vi "thcd_visa_init.vi"(2 "err_in":errorcluster, 3 "Serial Settings:Baud Rate":u32(ring)=19200 items=["9.6KHz"=9600, "19.2KHz"=19200], 4 "thcd_visa":refnum<visa-resource-name>) -> (0 "err_out":errorcluster, 1 "thcd_visa":refnum<visa-resource-name>)   [LabVIEW 2018, in "1039_mod.lvlib"]
uses:
  <vilib>/Instr/_visa.llb/VISA Flush IO Buffer Mask.ctl
  1039_mod/1039_mod.lvlib
panel:
  in  "Mask":T1=64 items=["Flush Receive Buffer"=16, "Write Transmit Buffer to Device"=32, "Flush Receive Buffer (No I/O)"=64, "Flush Transmit Buffer"=128]
  in  "Message Based Settings:Suppress End Enable":bool
  in  "Message Based Settings:Send End Enable":bool=TRUE
  in  "Message Based Settings:Termination Character Enable":bool=TRUE
  in  "Serial Settings:End Mode for Writes":u16(ring)=2 items=["None", "Last Bit", "TermChar", "Break"]
  in  "Serial Settings:End Mode for Reads":u16(ring)=2 items=["None", "Last Bit", "TermChar"]
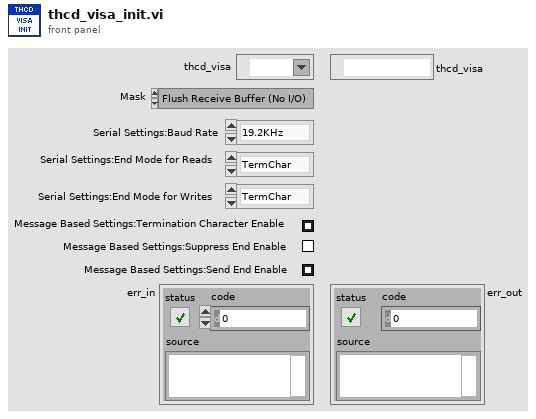
[diagram p1: front panel]
types:
  T1 = typedef "VISA Flush IO Buffer Mask.ctl" = u16
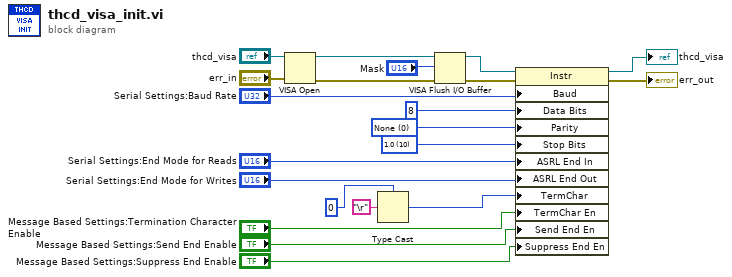
[diagram p0: block diagram]
diagram:
  w18 = u16 10 items=["1.0"=10, "1.5"=15, "2.0"=20] ("Serial Settings:Stop Bits")
  w19 = u16 0 items=["None", "Odd", "Even", "Mark", "Space"] ("Serial Settings:Parity")
  n1 = VISA Open(error in (no error)="err_in", VISA resource name="thcd_visa") -> (VISA resource name=w8:refnum<visa-resource-name>, error out=w7:errorcluster)  [unwired: 3 in]
  n2 = Type Cast(type=u8 0, x="\r") -> (*(type *) &x=w10:u8)
  n3 = VISA Flush I/O Buffer(VISA resource name=w8, mask (16)="Mask", error in (no error)=w7) -> (VISA resource name out=w5:refnum<visa-resource-name>, error out=w6:errorcluster)
  n4 = property class="Instr"(reference=w5, error in=w6, "Baud"="Serial Settings:Baud Rate", "Data Bits"=u16 8 ("Serial Settings:Data Bits"), "Parity"=w19, "Stop Bits"=w18, "ASRL End In"="Serial Settings:End Mode for Reads", "ASRL End Out"="Serial Settings:End Mode for Writes", "TermChar"=w10, "TermChar En"="Message Based Settings:Termination Character Enable", "Send End En"="Message Based Settings:Send End Enable", "Suppress End En"="Message Based Settings:Suppress End Enable") -> (reference out=→"thcd_visa":refnum<visa-resource-name>, error out=→"err_out":errorcluster)
